vi "Read Resolution.vi"(8 "Error in":errorcluster, 11 "Device in":refnum<class "Device.lvclass">) -> (0 "Error out":errorcluster, 2 "Resolution":dbl, 3 "Device out":refnum<class "Device.lvclass">)   [LabVIEW 2020, in "Device.lvclass"]
uses:
  Device.lvclass
  Device.lvclass/Device.ctl
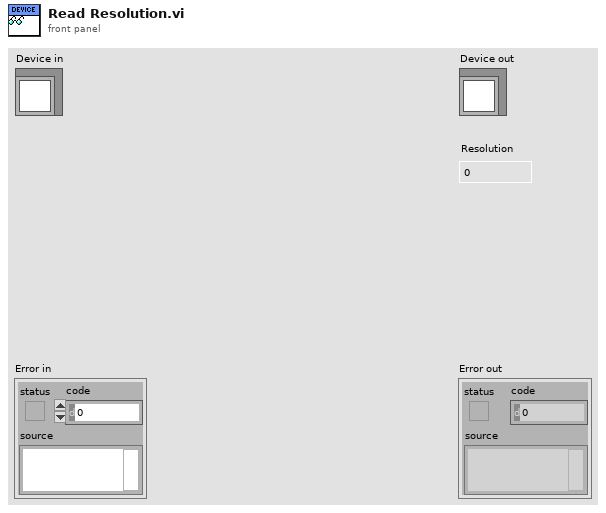
[diagram p1: front panel]
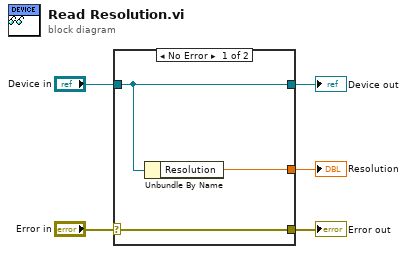
[diagram p0: block diagram]
diagram:
  n1 = case shown="No Error" "Error in" {
    selector: "Error in" -> [w8 w9]
    tunnel: [w8 w9] -> w4
    tunnel: [w7 w10] -> w2
    tunnel: "Device in" -> [w7 w10]
    tunnel: [w6 _] -> w1
    frame No Error {
      n2 = Unbundle By Name(w7) -> ("Resolution"=w6:dbl)
    }
    frame Error {
    }
  }
  "Error out" <- w4
  "Device out" <- w2
  "Resolution" <- w1
